vi "Extract.vi"(6 "TracesWrite error":errorcluster, 8 "VI folder":path, 9 "Extract path":path, 10 "Pixmap.bin path":path, 11 "Traces.txt path":path) -> (2 "Extract.c error":string, 3 "stdout":string, 4 "Extract error":errorcluster)   [LabVIEW 2023]
panel:
  in  "User interface":T1(tab)
  in  "User entries":enum32{""}(tab)
  in  "Customization":enum32{"Customization"}(tab)
  in  "Colors":enum32{"Colors"}(tab)
  in  "Size":enum32{"Size"}(tab)
  in  "Loop FOR 1":enum32{"Loop FOR 1"}(tab)
  in  "Arrays":enum32{"Arrays"}(tab)
  in  "Script.m":enum32{"Script.m"}(tab)
  in  "Extract.c output string scan":enum32{"Extract.c output string scan"}(tab)
  in  "T: tt1 tt2 tt3 ...":enum32{"T: tt1 tt2 tt3 ..."}(tab)
  in  "C: cc":enum32{"C: cc"}(tab)
  in  "Loop FOR 2":enum32{"Loop FOR 2"}(tab)
  out "Input arguments":string
  in  "LabVIEW":enum32{"LabVIEW"}(tab)
  in  "MATLAB":enum32{"MATLAB"}(tab)
  in  "C":enum32{"C"}(tab)
  in  "MATLAB":enum32{"MATLAB"}(tab)
  in  "C":enum32{"C"}(tab)
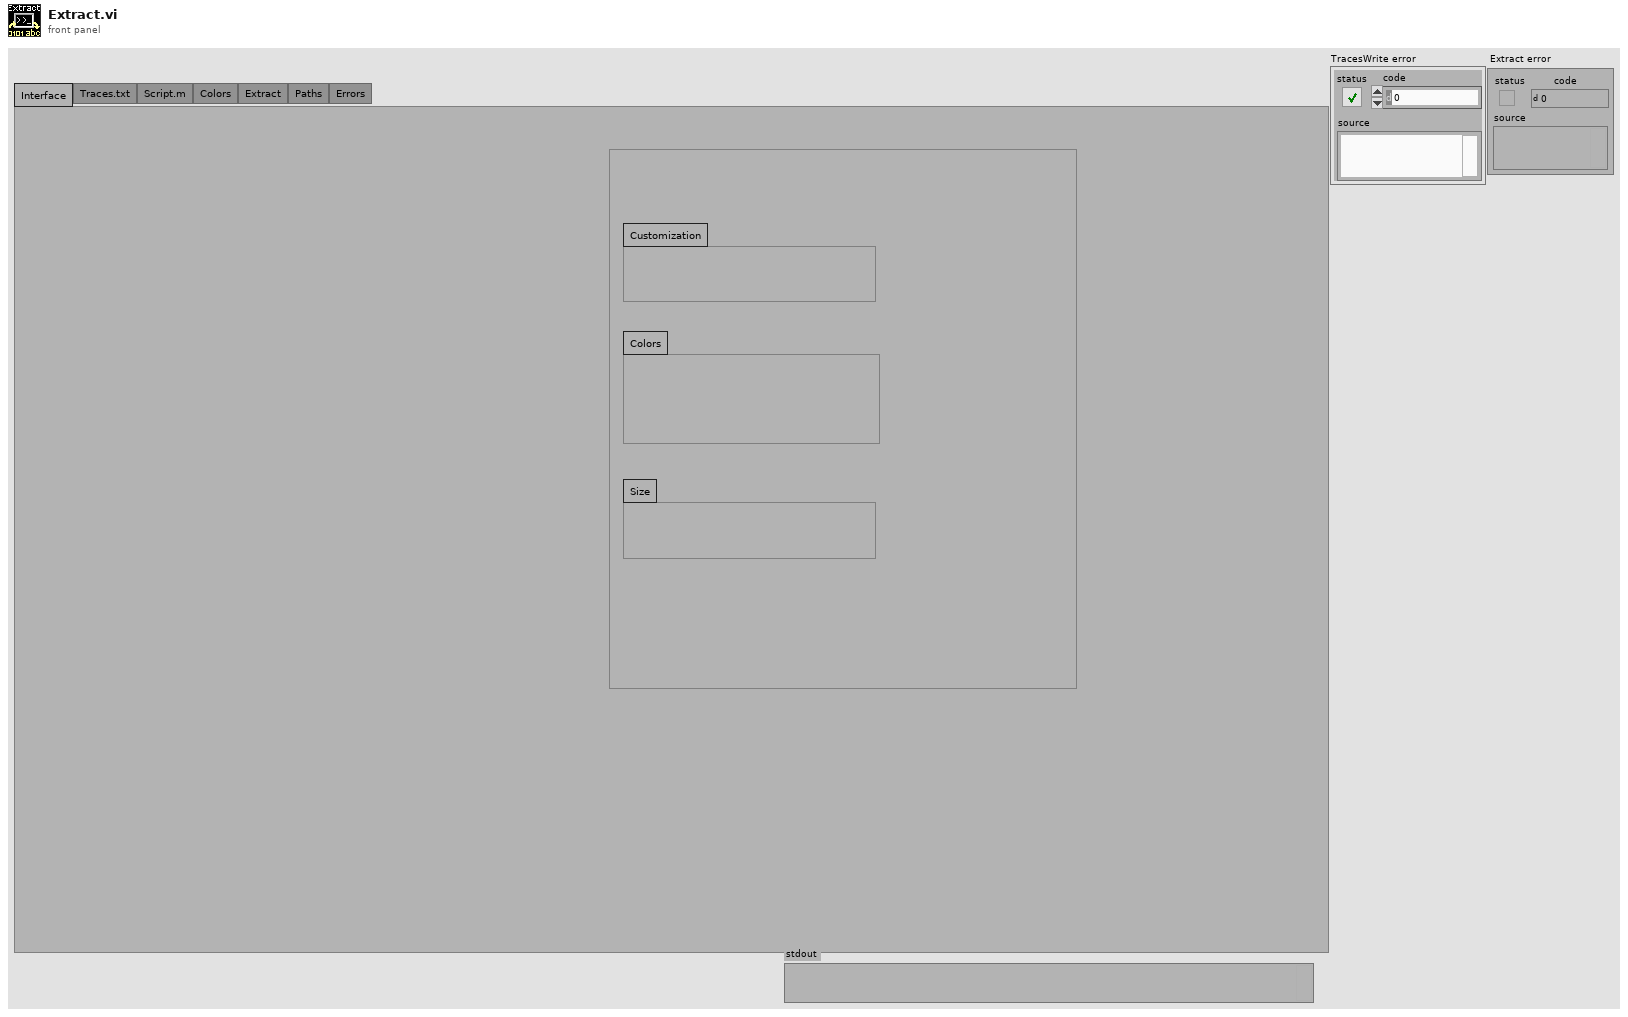
[diagram p1: front panel]
types:
  T1 = enum32{"Interface", "Traces.txt", "Script.m", "Colors", "Extract", "Paths", "Errors"}
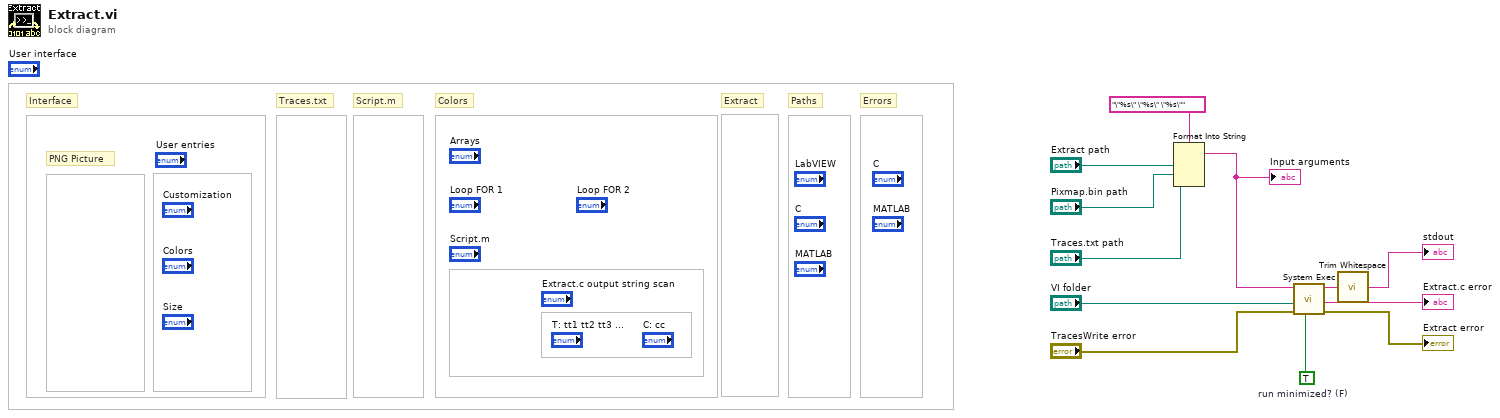
[diagram p0: block diagram]
diagram:
  w11 = TRUE  # run minimized? (F)
  # "PNG Picture"
  # "Errors"
  # "Paths"
  # "Extract"
  # "Colors"
  # "Script.m"
  # "Traces.txt"
  # "Interface"
  n1 = Format Into String(format string="\"%s\" \"%s\" \"%s\"", "Extract path", "Pixmap.bin path", "Traces.txt path") -> (resulting string=w6:string)  [unwired: 2 in, 1 out]
  "Input arguments" <- w6
  n2 = call <vilib>:"System Exec.vi"("run minimized? (F)"=w11, "error in (no error)"="TracesWrite error", "working directory"="VI folder", "command line"=w6) -> ("error out"=→"Extract error":errorcluster, "standard error"=→"Extract.c error":string, "standard output"=w2:string)  [unwired: 4 in, 1 out]
  n3 = call <vilib>:"Trim Whitespace.vi"("string"=w2) -> ("trimmed string"=→"stdout":string)  [unwired: 1 in]
